vi "类型3自动测试结果.vi"(8 "合格?":bool, 11 "第几组":i32) -> ()   [LabVIEW 2010]
uses:
  全局量/自动测试结果.vi
panel:
  # "自动测试类型3最终结论"
  # "1X80"
  # "自动测试类型3最终结论"
  # "1X80"
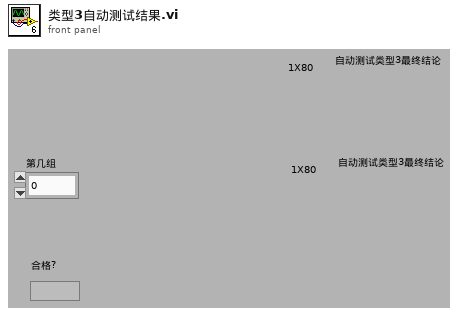
[diagram p1: front panel]
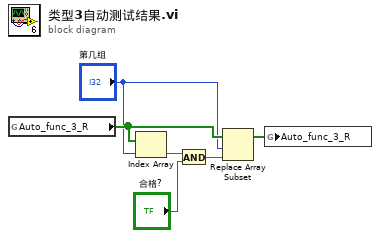
[diagram p0: block diagram]
diagram:
  n1 = global read "自动测试结果.vi" "Auto_func_3_R"() -> (w5:bool[])
  n2 = Index Array(array=w5, index="第几组") -> (element=w2:bool)
  n3 = And(x=w2, y="合格?") -> (x .and. y?=w4:bool)
  n4 = Replace Array Subset(array=w5, new element=w4, index="第几组") -> (w6:bool[])
  n5 = global write "自动测试结果.vi" "Auto_func_3_R"(w6) -> ()
